vi "PythontoArray.vi"(8 "error in (no error)":errorcluster, 10 "command line":string="python SkysparkBuild3.py", 11 "working directory":path=path "") -> (0 "error out":errorcluster, 2 "standard output":string, 3 "Output Array":string[][](array[string]))   [LabVIEW 2020]
uses:
  859b58b0-79df-43f2-a2e9-99a1650faf3a.vi
panel:
  out "Table Control":string[][](table)
  in  "format string":string
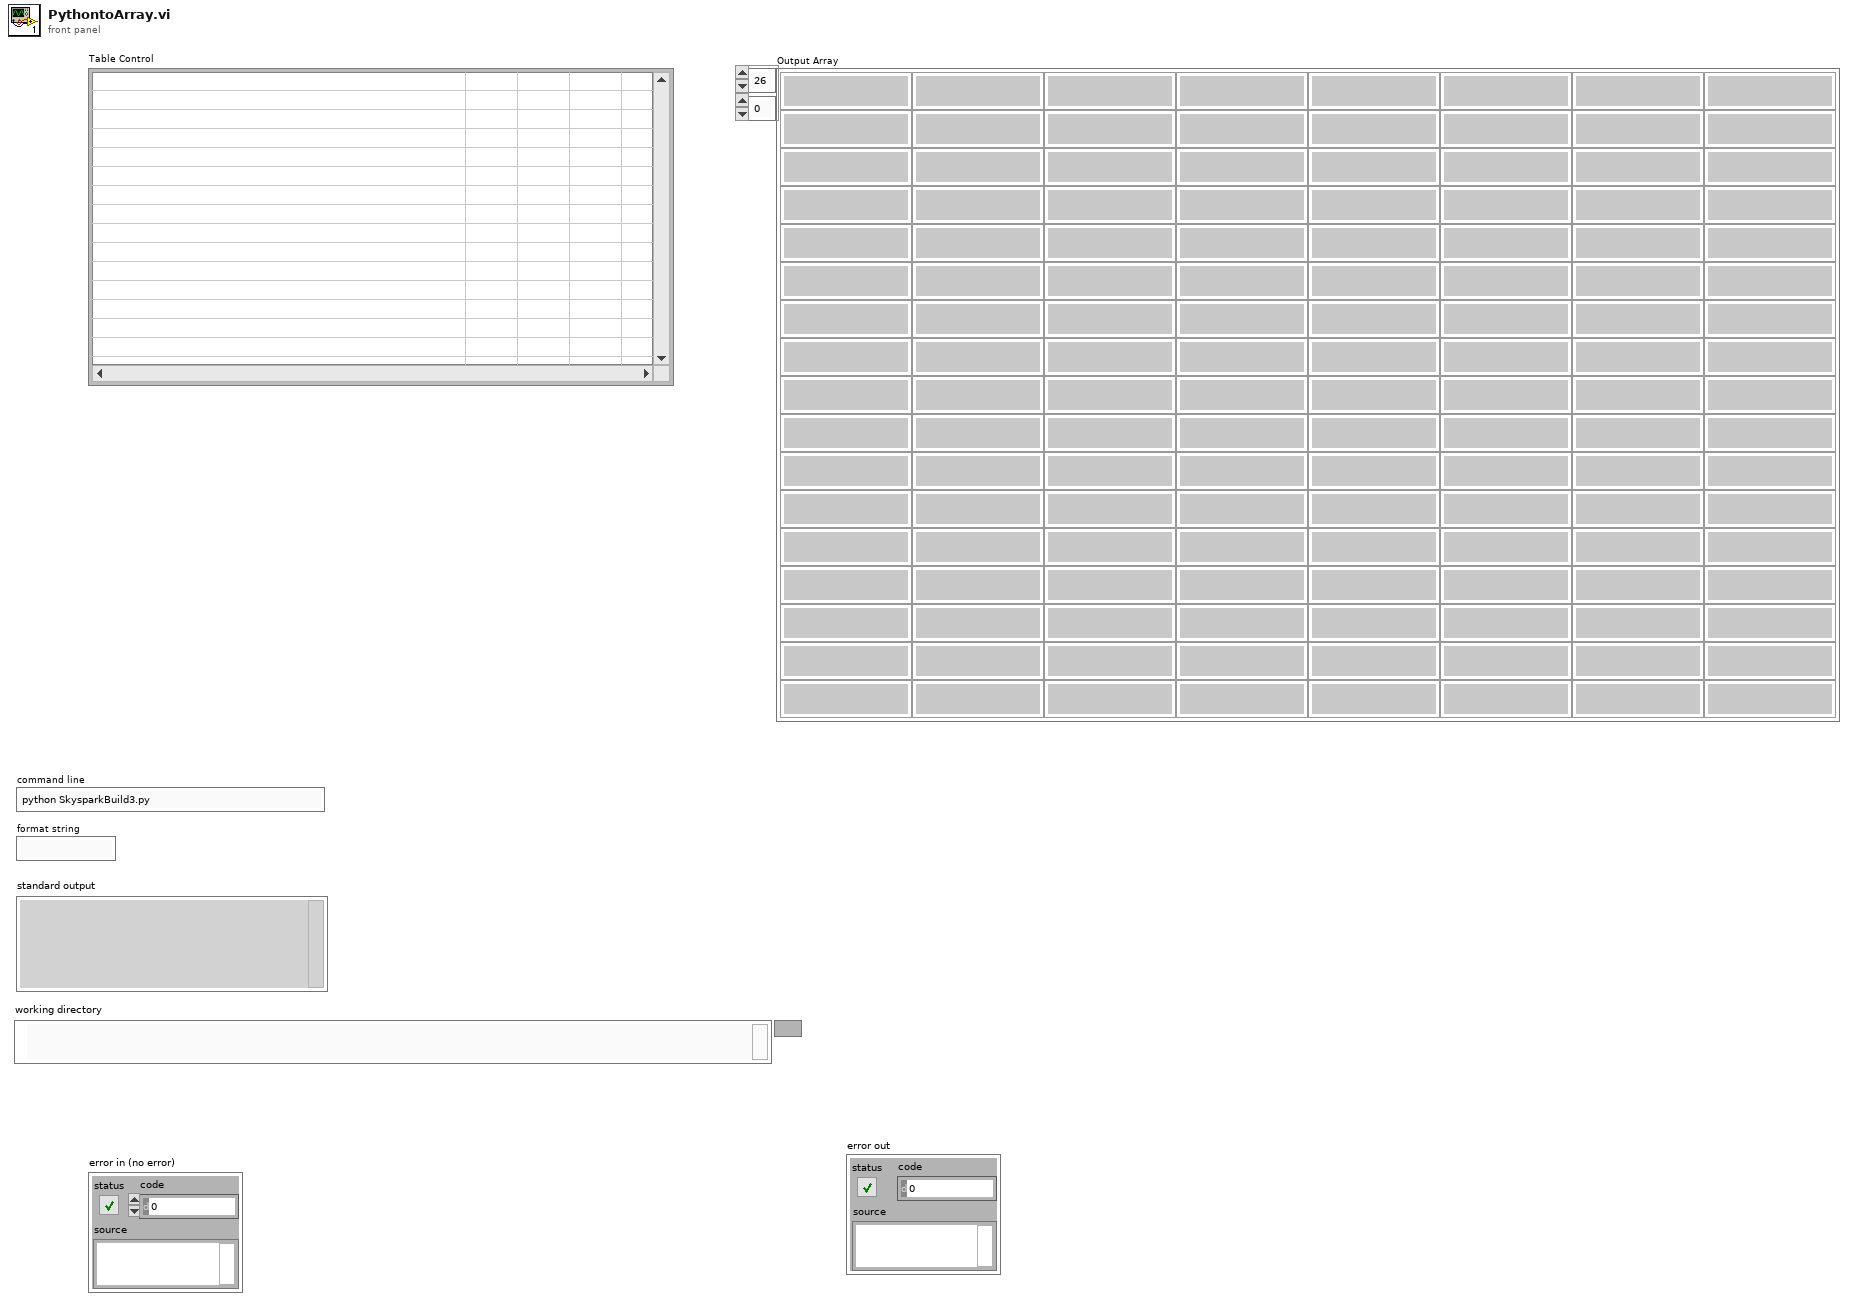
[diagram p1: front panel]
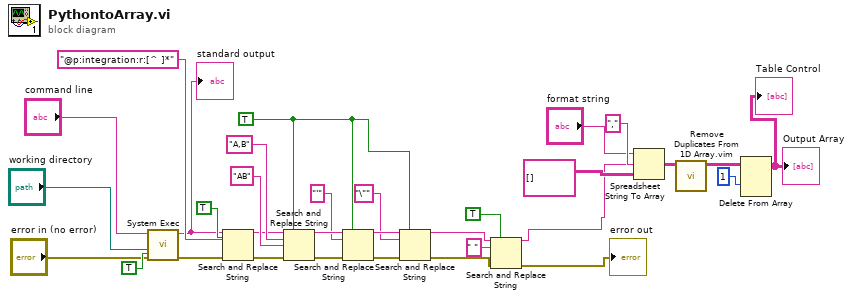
[diagram p0: block diagram]
diagram:
  w14 = TRUE ("replace all? (F)")
  n1 = call <vilib>:"System Exec.vi"("run minimized? (F)"=TRUE, "error in (no error)"="error in (no error)", "working directory"="working directory", "command line"="command line") -> ("error out"=w10:errorcluster, "standard output"=w18:string)  [unwired: 4 in, 2 out]
  "standard output" <- w18
  n2 = Search and Replace String(replace all?=TRUE ("replace all? (F)"), input string=w18, search string="@p:integration:r:[^ ]*", error in=w10) -> (result string=w19:string, error out=w9:errorcluster)  [unwired: 4 in, 2 out]
  n3 = Search and Replace String(replace all?=w14, input string=w19, search string="A,B" ("substring (\"\")"), replace string="AB" ("replace string (\"\")"), error in=w9) -> (result string=w17:string, error out=w8:errorcluster)  [unwired: 3 in, 2 out]
  n4 = Search and Replace String(replace all?=w14, input string=w17, search string="'", error in=w8) -> (result string=w16:string, error out=w15:errorcluster)  [unwired: 4 in, 2 out]
  n5 = Search and Replace String(replace all?=w14, input string=w16, search string="\"", error in=w15) -> (result string=w3:string, error out=w6:errorcluster)  [unwired: 4 in, 2 out]
  n6 = Search and Replace String(replace all?=TRUE ("replace all? (F)"), input string=w3, search string=" ", error in=w6) -> (result string=w2:string, error out=→"error out":errorcluster)  [unwired: 4 in, 2 out]
  n7 = Spreadsheet String To Array(delimiter (Tab)=",", format string="format string", spreadsheet string=w2, array type (2D Dbl)=string[][] []) -> (array=w26:string[][])
  n8 = call "Remove Duplicates From 1D Array.vim"("array"=w26) -> ("array with duplicates removed"=w25:string[][])  [unwired: 10 in]
  n9 = Delete From Array(array=w25, index (row)=1) -> (array with subset deleted=→"Output Array" →"Table Control":string[][])  [unwired: 2 in, 1 out]
